vi "minicryo_RT&RH_202102.vi"() -> ()   [LabVIEW 2013]
uses:
  <vilib>/Analysis/baseanly.llb/Mean (DBL).vi
  subVI/DeltaRamp_globals.vi
  subVI/B_Globals.vi
  subVI/Global 2.vi
  <vilib>/Analysis/NI_AALBase.lvlib
panel:
  out "Armed?":string="1\n"
  out "B_set [T]":dbl=0.05
  in  "Reading Delay [ms]":i32=20 min=5
  in  "RW Delay":i32=5
  out "Exec Time [ms]":u32=103
  out "read buffer":string="+1.42638245E+01,+7.060E+04\n"
  in  "B/T":bool=TRUE
  in  "Smart Avs":bool=TRUE
  in  "Points":dbl=1.0
  out "PpP":dbl=3.0
  in  "Combo Box":string(combo)="Temp"
  in  "Save":bool
  in  "Abort Delta":bool
  out "B [T]":dbl=0.05028
  in  "Arm":bool
  in  "Measure":bool
  in  "Comp":dbl=10.0
  in  "Delay":dbl=0.0020000000000000018
  in  "I_Max":dbl=1e-05
  out "T":cluster{"X":dbl[], "Y":dbl[]}[](graph) caption="XY Graph"
  in  "Reset":bool
  out "Spl T [K]":dbl=3.68549
  out "R [Ohm]":dbl=14.2638245
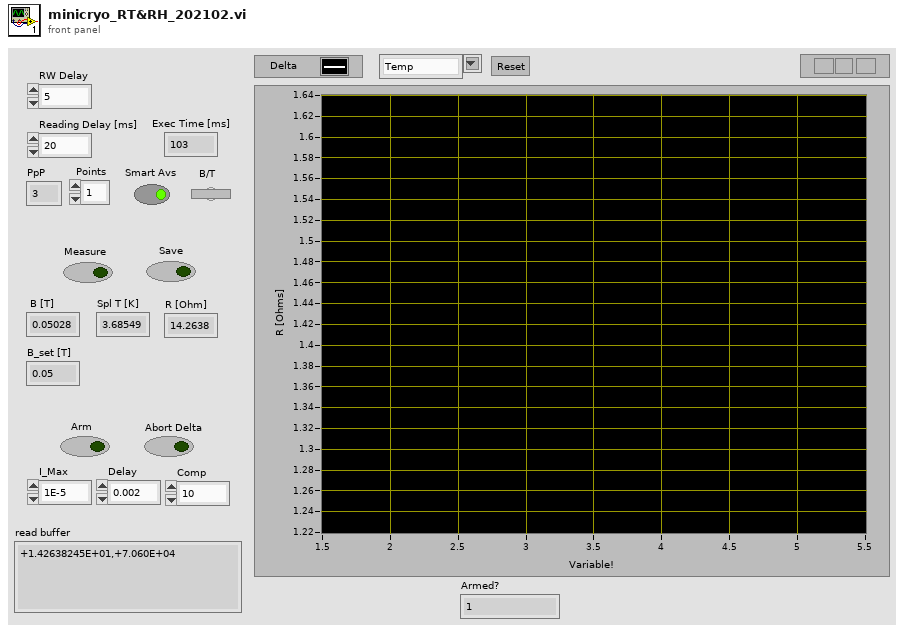
[diagram p1: front panel]
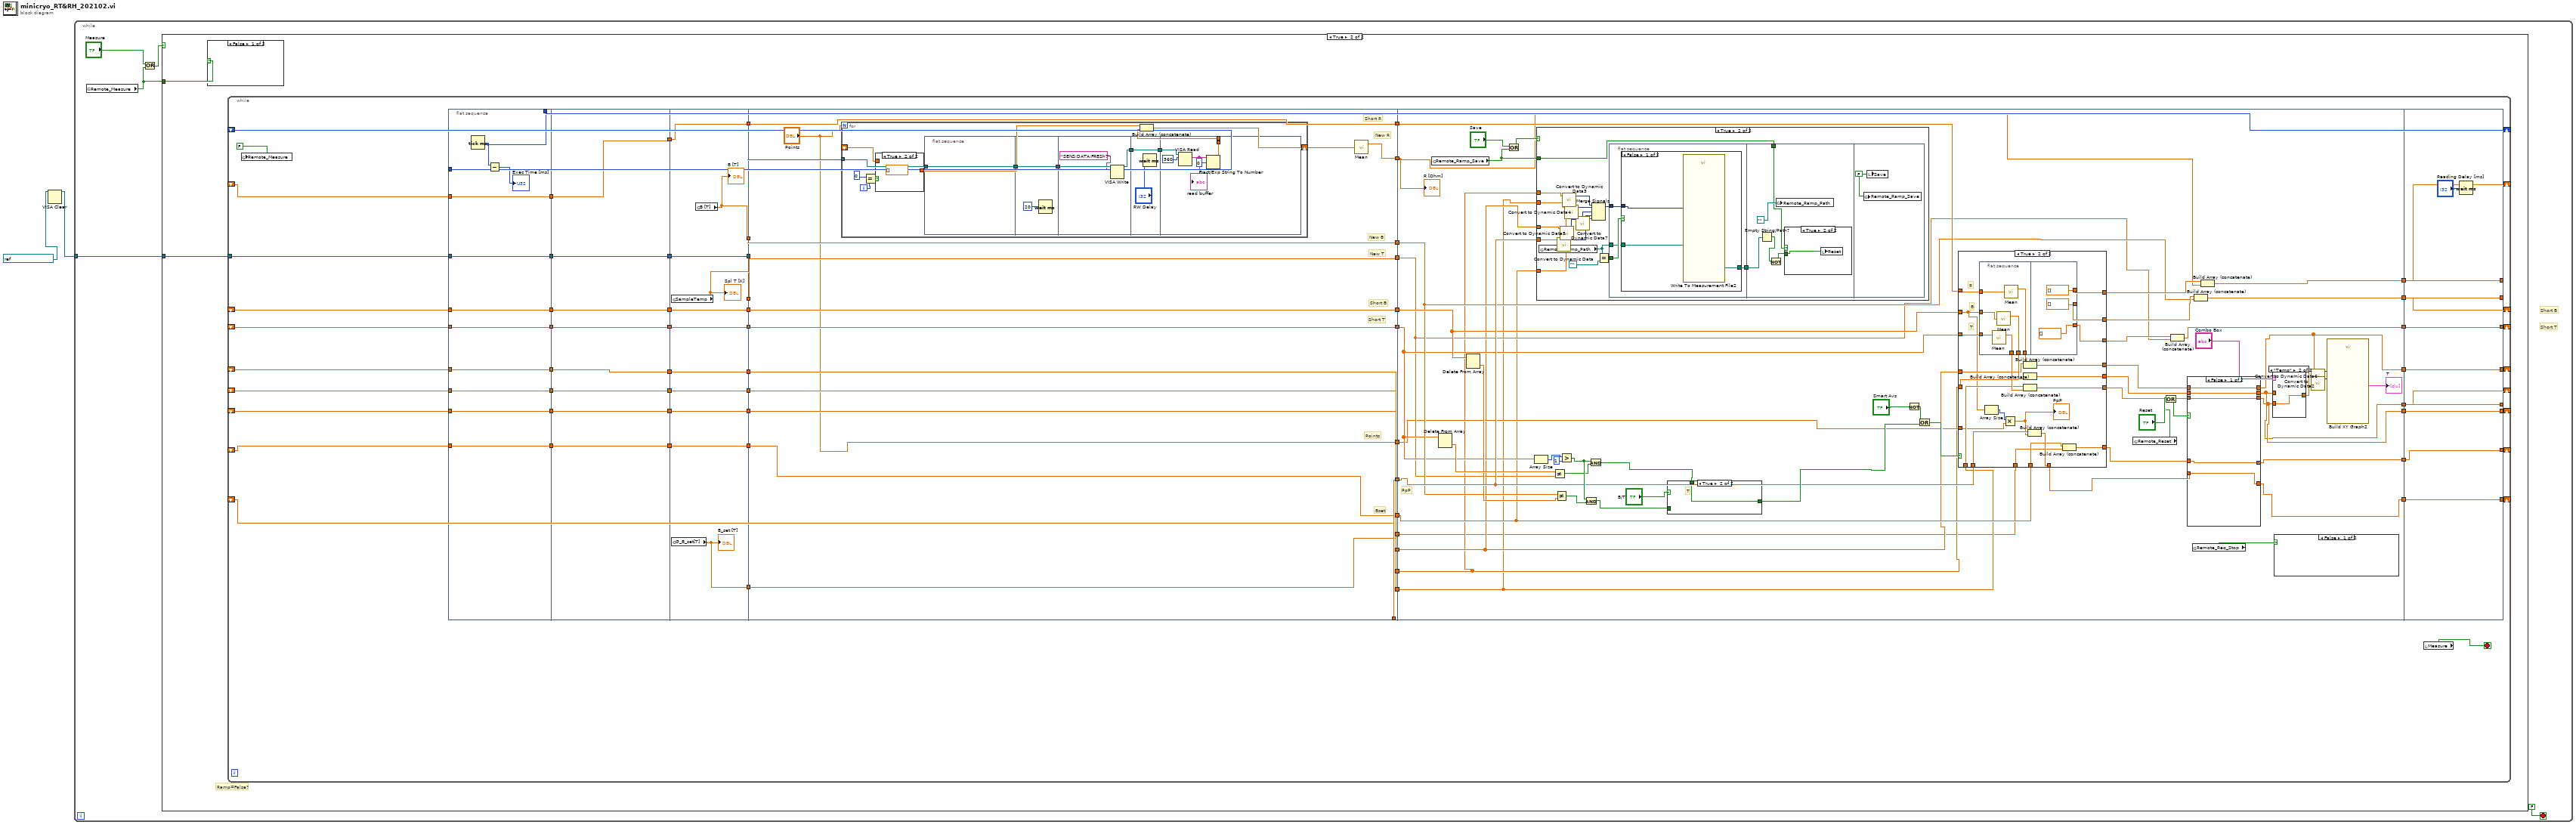
[diagram p0: block diagram]
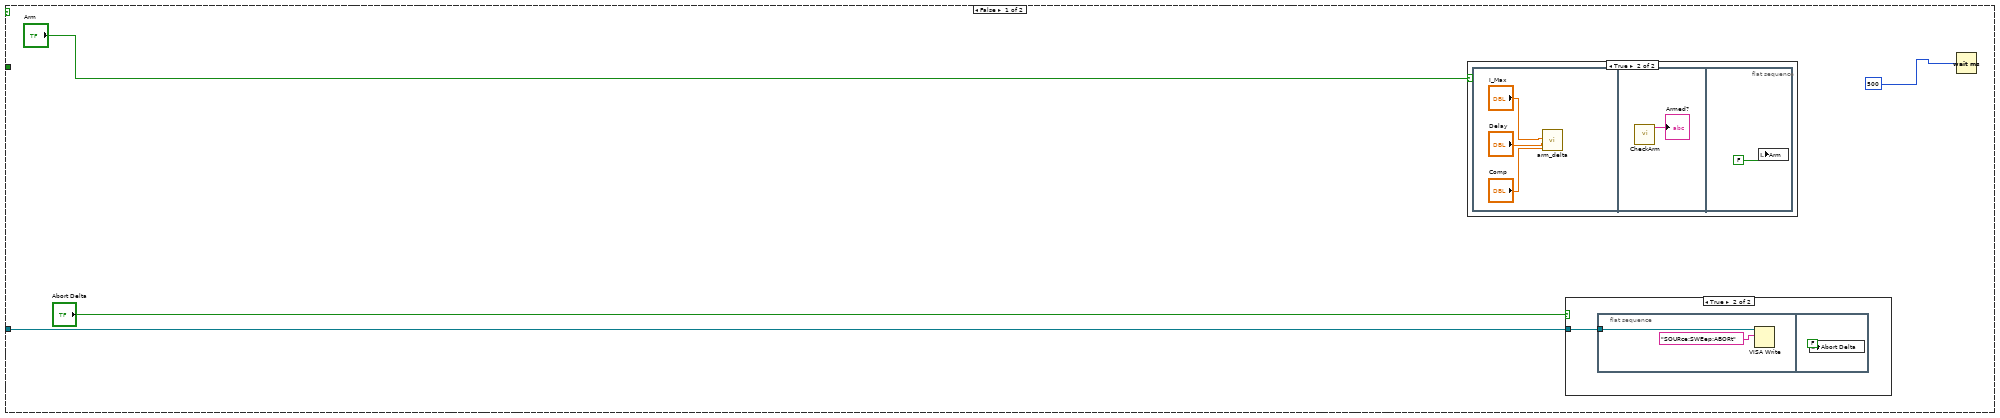
[diagram p2: hidden frame]
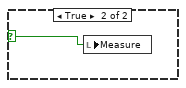
[diagram p5: hidden frame]
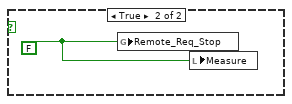
[diagram p8: hidden frame]
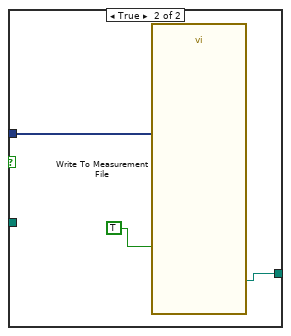
[diagram p12: hidden frame]
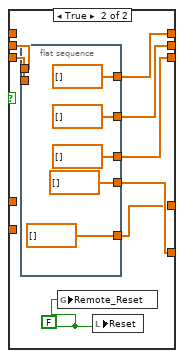
[diagram p14: hidden frame]
diagram:
  n1 = VISA Clear(VISA resource name=refnum<visa-resource-name> "GPIB0::20::INSTR" ("Keithley")) -> (VISA resource name out=w2:refnum<visa-resource-name>)  [unwired: 1 in, 1 out]
  n2 = while {
    tunnel: w2 -> [w6]
    stop <- FALSE stop-if-true
    # "Short T"
    # "Short B"
    n3 = global read "DeltaRamp_globals.vi" "Remote_Measure"() -> (w3:bool)
    n4 = Or(x="Measure", y=w3) -> (x .or. y?=w5:bool)
    n5 = case shown="True" w5 {
      tunnel: w6 -> [w9 w22]
      tunnel: w3 -> [_ w21]
      frame False {
        n6 = case shown="True" "Arm" {
          frame False {
          }
          frame True {
            n7 = flat-sequence {
              frame #0 {
                n8 = call "arm_delta.vi"("Compliance [V]"="Comp", "DELAY [sec]"="Delay", "I-HIGH [A]"="I_Max") -> ()  [unwired: 9 in]
              }
              frame #1 {
                n9 = call "CheckArm.vi"() -> ("read buffer"=→"Armed?":string)  [unwired: 10 in, 1 out]
              }
              frame #2 {
                n10 = local write "Arm"(FALSE) -> ()
              }
            }
          }
        }
        n11 = case shown="True" "Abort Delta" {
          tunnel: w9 -> [_ w12]
          frame False {
          }
          frame True {
            n12 = flat-sequence {
              tunnel: w12 -> [w14]
              frame #0 {
                n13 = VISA Write(VISA resource name=w14, write buffer="SOURce:SWEep:ABORt") -> ()  [unwired: 1 in, 3 out]
              }
              frame #1 {
                n14 = local write "Abort Delta"(FALSE) -> ()
              }
            }
          }
        }
        n15 = Wait (ms)(milliseconds to wait=500) -> ()  [unwired: 1 out]
      }
      frame True {
        # "Ramp=False?"
        n16 = case shown="False" w21 {
          selector: w21 -> [_ w23]
          frame False {
          }
          frame True {
            n17 = local write "Measure"(w23) -> ()
          }
        }
        n18 = while {
          shift-right: [w43] -> _
          shift-left: _ -> [w50]
          shift-right: [w62] -> _
          shift-left: _ -> [w67]
          tunnel: w22 -> [w86]
          shift-right: [w60] -> _
          shift-left: _ -> [w73]
          shift-right: [w42] -> _
          shift-left: _ -> [w54]
          shift-right: [w44] -> _
          shift-left: _ -> [w59]
          shift-right: [w61] -> _
          shift-left: _ -> [w77]
          shift-right: [w87] -> _
          shift-left: _ -> [w88]
          shift-right: [w90] -> _
          shift-left: _ -> [w91]
          shift-right: [w26] -> _
          shift-left: _ -> [w31]
          stop <- w33 stop-if-true
          n19 = global write "DeltaRamp_globals.vi" "Remote_Measure"(FALSE) -> ()
          n20 = flat-sequence {
            tunnel: w91 -> [w103]
            tunnel: [w101] -> w90
            tunnel: w86 -> [w100]
            tunnel: [w100] -> w83
            tunnel: w77 -> [w99]
            tunnel: [w99] -> w76
            tunnel: w73 -> [w98]
            tunnel: [w98] -> w70
            tunnel: w67 -> [w97]
            tunnel: [w97] -> w65
            tunnel: w59 -> [w96]
            tunnel: [w96] -> w56
            tunnel: [w95] -> w55
            tunnel: w54 -> [w95]
            tunnel: [w94] -> w51
            tunnel: w50 -> [w94]
            tunnel: [w93] -> w32
            tunnel: w31 -> [w93]
            tunnel: [w111] -> w84
            tunnel: w83 -> [w111]
            tunnel: w76 -> [w110]
            tunnel: [w110] -> w75
            tunnel: [w109] -> w71
            tunnel: w70 -> [w109]
            tunnel: [w108] -> w66
            tunnel: w65 -> [w108]
            tunnel: [w107] -> w57
            tunnel: w56 -> [w107]
            tunnel: w55 -> [w106]
            tunnel: [w106] -> w52
            tunnel: w51 -> [w105]
            tunnel: [w105] -> w48
            tunnel: w32 -> [w104]
            tunnel: [w104] -> w29
            tunnel: [w122] -> w85
            tunnel: w84 -> [w122]
            tunnel: [w121] -> w81
            tunnel: [w120] -> w79
            tunnel: w75 -> [w119]
            tunnel: [w119] -> w74
            tunnel: [w118] -> w72
            tunnel: w71 -> [w118]
            tunnel: w66 -> [w117]
            tunnel: [w117] -> w64
            tunnel: [w116] -> w58
            tunnel: w57 -> [w116]
            tunnel: [w115] -> w53
            tunnel: w52 -> [w115]
            tunnel: [w114] -> w49
            tunnel: w48 -> [w114]
            tunnel: [w113] -> w30
            tunnel: w29 -> [w113]
            tunnel: [w112] -> w25
            tunnel: [w136] -> w89
            tunnel: w88 -> [w136]
            tunnel: w85 -> [w135]
            tunnel: [w134] -> w82
            tunnel: w81 -> [w133]
            tunnel: [w133] -> w80
            tunnel: w79 -> [w132]
            tunnel: [w132] -> w78
            tunnel: w74 -> [w131]
            tunnel: w72 -> [w130]
            tunnel: [w131] -> w69
            tunnel: [w130] -> w68
            tunnel: w64 -> [w129]
            tunnel: [w129] -> w63
            tunnel: w58 -> [w128]
            tunnel: w53 -> [w127]
            tunnel: w49 -> [w126]
            tunnel: [w128] -> w47
            tunnel: [w127] -> w46
            tunnel: [w126] -> w45
            tunnel: ["Points"] -> w41
            tunnel: w30 -> [w124]
            tunnel: [w124] -> w28
            tunnel: w25 -> [w123]
            tunnel: [w123] -> w24
            tunnel: w89 -> [w193]
            tunnel: w82 -> [w185]
            tunnel: w80 -> [w184]
            tunnel: w78 -> [w180]
            tunnel: w69 -> [w189]
            tunnel: w68 -> [w183]
            tunnel: w63 -> [w188]
            tunnel: w47 -> [w168]
            tunnel: w46 -> [w167]
            tunnel: w45 -> [w166]
            tunnel: w41 -> [w172]
            tunnel: [w173] -> w40
            tunnel: [w186] -> w39
            tunnel: [w182] -> w38
            tunnel: [w181] -> w37
            tunnel: [w179] -> w36
            tunnel: [w175] -> w35
            tunnel: [w174] -> w34
            tunnel: w28 -> [w169]
            tunnel: [w171] -> w27
            tunnel: w24 -> [w165]
            tunnel: [w318] -> w42
            tunnel: [w319] -> w43
            tunnel: [w320] -> w44
            tunnel: [w321] -> w60
            tunnel: [w322] -> w61
            tunnel: [w323] -> w62
            tunnel: [w324] -> w87
            tunnel: w40 -> [w324]
            tunnel: w39 -> [w323]
            tunnel: w38 -> [w322]
            tunnel: w37 -> [w321]
            tunnel: w36 -> [w320]
            tunnel: w35 -> [w319]
            tunnel: w34 -> [w318]
            tunnel: w27 -> [w316]
            tunnel: [w316] -> w26
            frame #0 {
              n21 = Tick Count (ms)() -> (millisecond timer value=w101:u32)
              n22 = Subtract(x=w101, y=w103) -> (x-y=→"Exec Time [ms]":u32)
            }
            frame #1 {
            }
            frame #2 {
              n23 = global read "Global 2.vi" "SampleTemp"() -> (w120:dbl)
              "Spl T [K]" <- w120
              n24 = global read "B_Globals.vi" "G_B_set[T]"() -> (w112:dbl)
              "B_set [T]" <- w112
              n25 = global read "B_Globals.vi" "B [T]"() -> (w121:dbl)
              "B [T]" <- w121
            }
            frame #3 {
              # "Bset"
              # "Points"
              # "Short R"
              # "New T"
              # "New B"
              # "Short T"
              # "Short B"
              # "New R"
              n26 = for {
                N: "Points" -> [_]
                tunnel: w135 -> [w149]
                shift-right: [w148] -> w137
                shift-left: _ -> [w140]
                i -> [w142]
                n27 = Equal?(x=0, y=w142) -> (x = y?=w144:bool)
                n28 = case shown="True" w144 {
                  tunnel: [w150 dbl[] [] ("Numeric")] -> w141
                  tunnel: w140 -> [w150 _]
                  frame False {
                  }
                  frame True {
                  }
                }
                n29 = flat-sequence {
                  tunnel: w149 -> [w152]
                  tunnel: [w152] -> w139
                  tunnel: w139 -> [w154]
                  tunnel: [w154] -> w138
                  tunnel: [w156] -> w145
                  tunnel: w138 -> [w157]
                  tunnel: [w158] -> w146
                  tunnel: w145 -> [w158]
                  tunnel: w146 -> [w161]
                  tunnel: [w162] -> w147
                  tunnel: [w162] -> _
                  frame #0 {
                  }
                  frame #1 {
                    n30 = Wait (ms)(milliseconds to wait=20) -> ()  [unwired: 1 out]
                  }
                  frame #2 {
                    n31 = VISA Write(VISA resource name=w157, write buffer="SENS:DATA:FRESh?" ("write buffer 2")) -> (VISA resource name out=w156:refnum<visa-resource-name>)  [unwired: 1 in, 2 out]
                  }
                  frame #3 {
                    n32 = Wait (ms)(milliseconds to wait="RW Delay") -> ()  [unwired: 1 out]
                  }
                  frame #4 {
                    n33 = VISA Read(VISA resource name=w161, byte count=u32 360) -> (read buffer=w160:string)  [unwired: 1 in, 3 out]
                    "read buffer" <- w160
                    n34 = Fract/Exp String To Number(string=w160, offset=0) -> (number=w162:dbl)  [unwired: 3 out]
                  }
                }
                n35 = Build Array (concatenate)(w141, w147) -> (w148:dbl[])
              }
              n36 = call-poly <vilib>:"Mean.vi"("X"=w137) -> ("mean"=w134:dbl)  [unwired: 1 out]
            }
            frame #4 {
              # "PpP"
              n37 = global read "DeltaRamp_globals.vi" "Remote_Ramp_Save"() -> (w205:bool)
              n38 = Delete From Array(array=w183) -> (deleted portion=w191:dbl)  [unwired: 2 in, 1 out]
              n39 = Delete From Array(array=w189) -> (deleted portion=w190:dbl)  [unwired: 2 in, 1 out]
              n40 = Or(x="Save", y=w205) -> (x .or. y?=w200:bool)
              n41 = Array Size(array=w183) -> (size(s)=w210:i32)
              n42 = case shown="True" w200 {
                tunnel: w205 -> [_ w272]
                tunnel: w193 -> [_ w271]
                tunnel: w169 -> [_ w266]
                tunnel: w168 -> [_ w269]
                tunnel: w167 -> [_ w268]
                tunnel: w166 -> [_ w267]
                frame False {
                }
                frame True {
                  n43 = global read "DeltaRamp_globals.vi" "Remote_Ramp_Path"() -> (w274:path)
                  n44 = call "Convert to Dynamic Data"("Array"=w271) -> ("Dynamic Data Type"=w270:dynamicdata)  [unwired: 3 in]
                  n45 = call "Convert to Dynamic Data5"("Array"=w269) -> ("Dynamic Data Type"=w277:dynamicdata)  [unwired: 3 in]
                  n46 = call "Convert to Dynamic Data3"("Array"=w268) -> ("Dynamic Data Type"=w279:dynamicdata)  [unwired: 3 in]
                  n47 = call "Convert to Dynamic Data4"("Array"=w267) -> ("Dynamic Data Type"=w278:dynamicdata)  [unwired: 3 in]
                  n48 = call "Convert to Dynamic Data7"("Array"=w266) -> ("Dynamic Data Type"=w265:dynamicdata)  [unwired: 3 in]
                  n49 = Merge Signals(w279, w278, w277, w270, w265) -> (w280:dynamicdata)
                  n50 = Equal?(x=w274, y=path "") -> (x = y?=w275:bool)
                  n51 = flat-sequence {
                    tunnel: w280 -> [w284]
                    tunnel: w275 -> [w283]
                    tunnel: w274 -> [w282]
                    tunnel: [w281] -> w273
                    tunnel: w273 -> [w293]
                    tunnel: w272 -> [w294]
                    frame #0 {
                      n52 = case shown="False" w283 {
                        tunnel: w284 -> [w287 w289]
                        tunnel: w282 -> [w286 _]
                        tunnel: [w285 w288] -> w281
                        frame False {
                          n53 = call "Write To Measurement File2"("Signals"=w287, "Filename"=w286) -> ("Filename Out"=w285:path)  [unwired: 15 in, 2 out]
                        }
                        frame True {
                          n54 = call "Write To Measurement File"("Signals"=w289, "Reset"=TRUE) -> ("Filename Out"=w288:path)  [unwired: 15 in, 2 out]
                        }
                      }
                    }
                    frame #1 {
                      n55 = Empty String/Path?(string/path=w293) -> (empty?=w292:bool)
                      n56 = Not(x=w292) -> (.not. x?=w291:bool)
                      n57 = global write "DeltaRamp_globals.vi" "Remote_Ramp_Path"(path "") -> ()
                      n58 = case shown="True" w294 {
                        tunnel: w291 -> [_ w296]
                        frame False {
                        }
                        frame True {
                          n59 = local write "Reset"(w296) -> ()
                        }
                      }
                    }
                    frame #2 {
                      w297 = FALSE
                      n60 = global write "DeltaRamp_globals.vi" "Remote_Ramp_Save"(w297) -> ()
                      n61 = local write "Save"(w297) -> ()
                    }
                  }
                }
              }
              n62 = Not Equal?(x=w191, y=w180) -> (x != y?=w211:bool)
              n63 = Not Equal?(x=w184, y=w190) -> (x != y?=w214:bool)
              n64 = Greater?(x=w210, y=1) -> (0:w213:bool)
              n65 = And(x=w213, y=w214) -> (x .and. y?=w215:bool)
              n66 = And(x=w213, y=w211) -> (x .and. y?=w216:bool)
              n67 = case shown="True" "B/T" {
                tunnel: w215 -> [w220 _]
                tunnel: w216 -> [_ w221]
                tunnel: [w220 w221] -> w217
                frame False {
                  # "B"
                }
                frame True {
                  # "T"
                }
              }
              n68 = Not(x="Smart Avs") -> (.not. x?=w207:bool)
              n69 = Or(x=w207, y=w217) -> (x .or. y?=w208:bool)
              n70 = case shown="True" w208 {
                tunnel: [w229 w253] -> w219
                tunnel: [w227 w252] -> w187
                tunnel: [w228 w239] -> w218
                tunnel: [w224 w250] -> w196
                tunnel: [w226 w249] -> w197
                tunnel: [w225 w247] -> w198
                tunnel: [w230 w245] -> w192
                tunnel: w193 -> [w230 w244]
                tunnel: w189 -> [w229 w235]
                tunnel: w183 -> [w228 w240]
                tunnel: w188 -> [w227 w241]
                tunnel: w168 -> [w226 w238]
                tunnel: w167 -> [w224 w237]
                tunnel: w166 -> [w225 w236]
                tunnel: w172 -> [_ w234]
                tunnel: w169 -> [w223 w233]
                tunnel: [w223 w232] -> w170
                tunnel: w165 -> [_ w231]
                frame False {
                }
                frame True {
                  # "T"
                  # "B"
                  # "R"
                  n71 = flat-sequence {
                    tunnel: [w258] -> w251
                    tunnel: [w257] -> w246
                    tunnel: [w259] -> w248
                    tunnel: w241 -> [w256]
                    tunnel: w235 -> [w255]
                    tunnel: w240 -> [w254]
                    tunnel: [dbl[] []] -> w239
                    tunnel: [dbl[] []] -> w253
                    tunnel: [dbl[] []] -> w252
                    frame #0 {
                      n72 = call-poly <vilib>:"Mean.vi"("X"=w254) -> ("mean"=w259:dbl)  [unwired: 1 out]
                      n73 = call-poly <vilib>:"Mean.vi"("X"=w255) -> ("mean"=w258:dbl)  [unwired: 1 out]
                      n74 = call-poly <vilib>:"Mean.vi"("X"=w256) -> ("mean"=w257:dbl)  [unwired: 1 out]
                    }
                    frame #1 {
                    }
                  }
                  n75 = Array Size(array=w235) -> (size(s)=w243:i32)
                  n76 = Multiply(x=w243, y=w234) -> (x*y=w242:dbl)
                  "PpP" <- w242
                  n77 = Build Array (concatenate)(w238, w246) -> (w249:dbl[])
                  n78 = Build Array (concatenate)(w237, w251) -> (w250:dbl[])
                  n79 = Build Array (concatenate)(w236, w248) -> (w247:dbl[])
                  n80 = Build Array (concatenate)(w244, w242) -> (w245:dbl[])
                  n81 = Build Array (concatenate)(w233, w231) -> (w232:dbl[])
                }
              }
              n82 = global read "DeltaRamp_globals.vi" "Remote_Reset"() -> (w201:bool)
              n83 = Or(x="Reset", y=w201) -> (x .or. y?=w203:bool)
              n84 = Build Array (concatenate)(w218, w180) -> (w181:dbl[])
              n85 = case shown="False" w203 {
                tunnel: w196 -> [w302 w310]
                tunnel: [w302 w309] -> w174
                tunnel: w198 -> [w301 w308]
                tunnel: [w301 w307] -> w175
                tunnel: [w300 w306] -> w179
                tunnel: w197 -> [w300 _]
                tunnel: [w299 w304] -> w173
                tunnel: w192 -> [w299 _]
                tunnel: [w298 w303] -> w171
                tunnel: w170 -> [w298 _]
                frame False {
                }
                frame True {
                  w305 = FALSE
                  n86 = flat-sequence {
                    tunnel: w310 -> [_]
                    tunnel: w308 -> [_]
                    tunnel: [dbl[] []] -> w307
                    tunnel: [dbl[] []] -> w309
                    tunnel: [dbl[] []] -> w306
                    tunnel: [dbl[] [] ("Numeric")] -> w304
                    tunnel: [dbl[] [] ("Numeric")] -> w303
                    frame #0 {
                    }
                  }
                  n87 = global write "DeltaRamp_globals.vi" "Remote_Reset"(w305) -> ()
                  n88 = local write "Reset"(w305) -> ()
                }
              }
              n89 = global read "DeltaRamp_globals.vi" "Remote_Req_Stop"() -> (w204:bool)
              n90 = Build Array (concatenate)(w219, w184) -> (w182:dbl[])
              n91 = Build Array (concatenate)(w187, w185) -> (w186:dbl[])
              n92 = case shown="\"Temp\"" "Combo Box" {
                tunnel: [w263 w264] -> w177
                tunnel: w175 -> [_ w264]
                tunnel: w174 -> [w263 _]
                frame "Field", Default {
                }
                frame "Temp" {
                }
              }
              n93 = case shown="False" w204 {
                frame False {
                }
                frame True {
                  w222 = FALSE
                  n94 = global write "DeltaRamp_globals.vi" "Remote_Req_Stop"(w222) -> ()
                  n95 = local write "Measure"(w222) -> ()
                }
              }
              n96 = call "Convert to Dynamic Data6"("Array"=w177) -> ("Dynamic Data Type"=w176:dynamicdata)  [unwired: 3 in]
              n97 = call "Convert to Dynamic Data2"("Array"=w179) -> ("Dynamic Data Type"=w178:dynamicdata)  [unwired: 3 in]
              n98 = call "Build XY Graph2"("Y Input"=w178, "X Input"=w176) -> ("XY Graph"=→"T":cluster{"X":dbl[], "Y":dbl[]}[])  [unwired: 8 in, 1 out]
              "R [Ohm]" <- w185
            }
            frame #5 {
              n99 = Wait (ms)(milliseconds to wait="Reading Delay [ms]") -> ()  [unwired: 1 out]
            }
          }
          n100 = local read "Measure"() -> (w33:bool)
        }
      }
    }
  }
